vi "Toggle TTL (SubVI).vi"(11 "Toggle?":bool) -> (3 "TTL Out":bool)   [LabVIEW 2014]
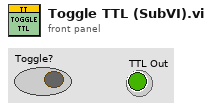
[diagram p1: front panel]
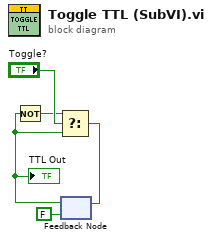
[diagram p0: block diagram]
diagram:
  n1 = feedback #1(FALSE ("Auto RESET")) -> (w4:bool)
  "TTL Out" <- w4
  n2 = Not(x=w4) -> (.not. x?=w3:bool)
  n3 = Select(t=w3, s="Toggle?", f=w4) -> (s? t:f=w2:bool)
  n4 = feedback-in #1(w2) -> ()
